vi "FGV Aufheizphase.vi"(0 "Status":T1, 7 "Error":bool, 9 "Aktiv/Inaktiv":u16, 11 "error in (no error)":errorcluster caption="Fehler (Eingang, kein Fehler)", 13 "Aktion":T2=enum."lesen") -> (4 "Aufheizphase":bool, 8 "Status":T1, 15 "error out":errorcluster caption="Fehler (Ausgang)")   [LabVIEW 2020, in "allgemeine Sub-VIs.lvlib"]
uses:
  allgemeine Sub-VIs.lvlib
  Aktion FGV Aufheizphase.ctl
  AufheizphaseCluster.ctl
  Funktionstasten/Funktionstasten-Aktion.ctl
  Funktionstasten/Zustaende.ctl
  Funktionstasten/Funktionstasten.lvlib
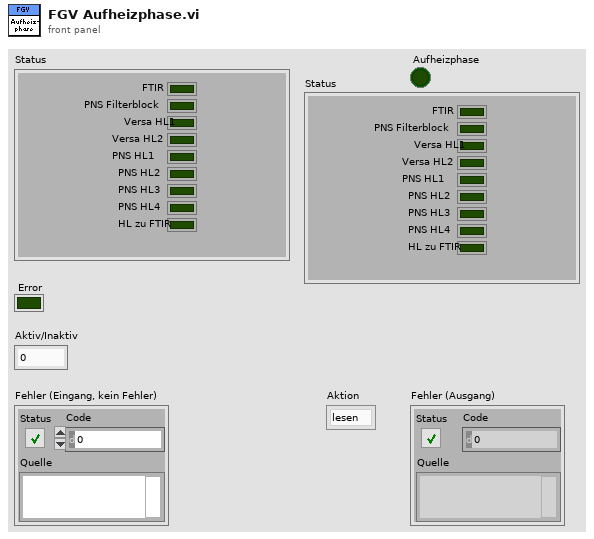
[diagram p1: front panel]
types:
  T1 = typedef "allgemeine Sub-VIs.lvlib/AufheizphaseCluster.ctl" = cluster{"FTIR":bool, "PNS Filterblock":bool, "Versa HL1":bool, "Versa HL2":bool, "PNS HL1":bool, "PNS HL2":bool, "PNS HL3":bool, "PNS HL4":bool, "HL zu FTIR":bool}
  T2 = typedef "allgemeine Sub-VIs.lvlib/Aktion FGV Aufheizphase.ctl" = enum16{"init", "lesen", "PNS Filterblock", "PNS HL1", "PNS HL2", "PNS HL3", "PNS HL4", "FTIR Messzelle", "HL 1", "HL 2", "HL zu FTIR", "auswerten"}
  T3 = typedef "Funktionstasten.lvlib/Zustaende.ctl" = enum16{"Standby", "Pause", "Eco", "Messen", "Kalibrieren", "Spülen Filter", "Spülen Leitung", "Umgebungsluft", "0-Gas", "Cal-Gas", "CG zu PNS", "-------------", "Init 1", "Init 2", "Init 3", "Init 4", "Messen vorbereiten", "Messen durchführen", "Exit"}
  T4 = typedef "Funktionstasten.lvlib/Funktionstasten-Aktion.ctl" = enum16{"Initialisieren", "Zustand setzen", "Taste gedrückt", "Fehler speichern", "Lesen", "Manuell", "Remote", "Bitparallel", "Samplepoint", "Zeit Prüfen", "reset Umschalten"}
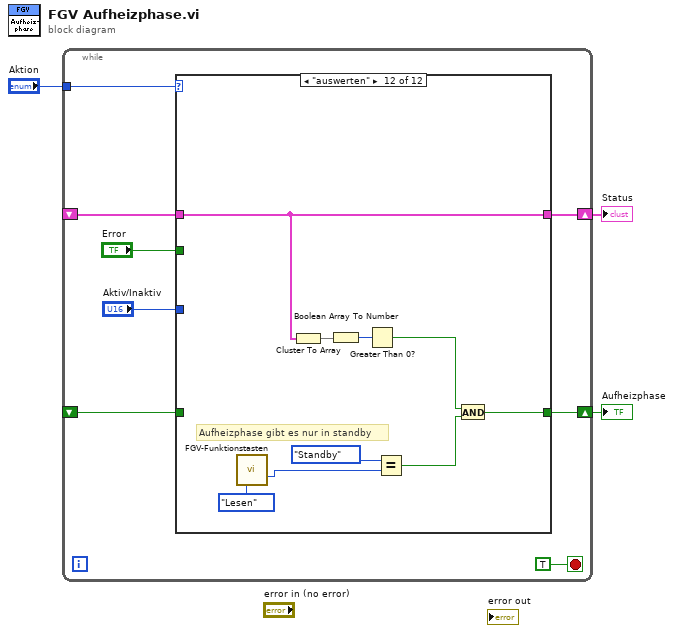
[diagram p0: block diagram]
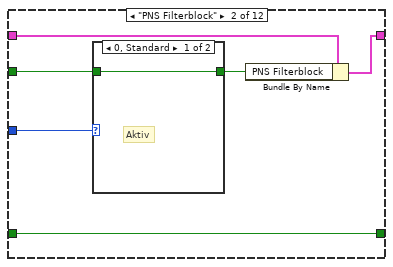
[diagram p3: hidden frame]
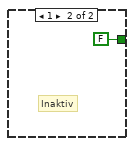
[diagram p4: hidden frame]
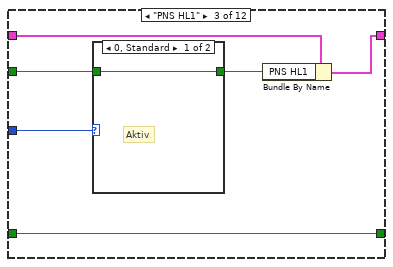
[diagram p5: hidden frame]
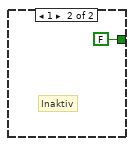
[diagram p6: hidden frame]
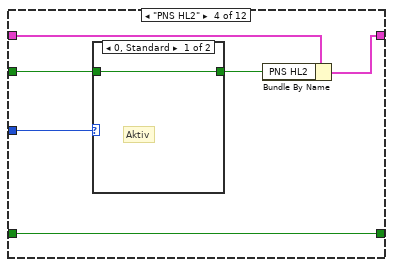
[diagram p7: hidden frame]
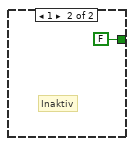
[diagram p8: hidden frame]
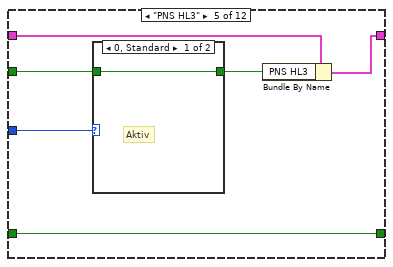
[diagram p9: hidden frame]
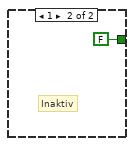
[diagram p10: hidden frame]
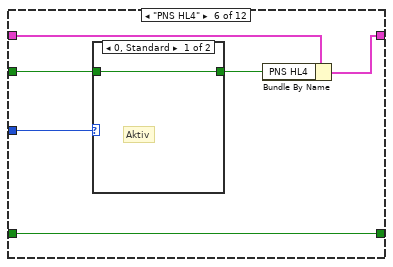
[diagram p11: hidden frame]
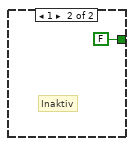
[diagram p12: hidden frame]
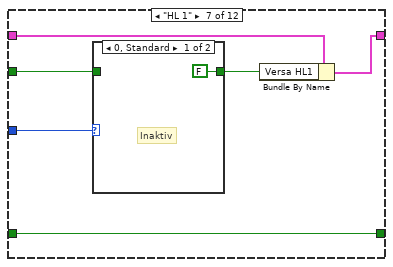
[diagram p13: hidden frame]
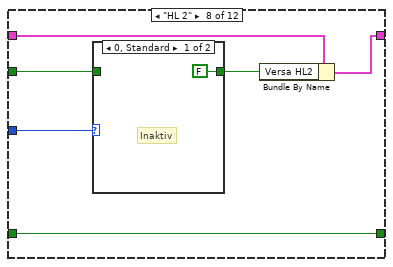
[diagram p15: hidden frame]
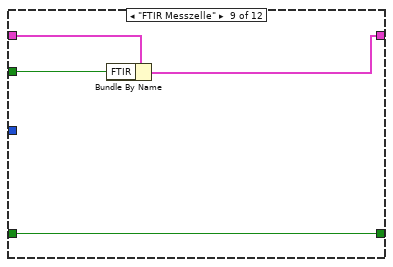
[diagram p17: hidden frame]
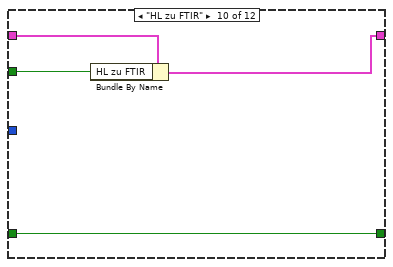
[diagram p18: hidden frame]
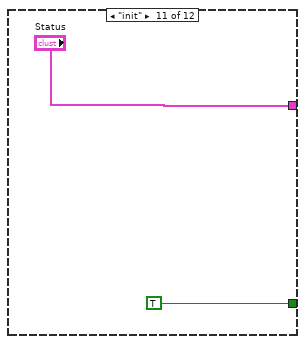
[diagram p19: hidden frame]
diagram:
  n1 = while {
    tunnel: "Aktion" -> [w10]
    shift-right: [w9] -> w1
    shift-left: _ -> [w8]
    shift-right: [w5] -> w2
    shift-left: _ -> [w4]
    stop <- TRUE stop-if-true
    n2 = case shown="\"auswerten\"" w10 {
      tunnel: [w13 w18 w26 w34 w42 w50 w58 w66 w72 w76 "Status" w88] -> w9
      tunnel: w8 -> [w13 w19 w27 w35 w43 w51 w59 w67 w73 w77 _ w88]
      tunnel: "Error" -> [_ w16 w24 w32 w40 w48 w56 w64 w71 w75 _ _]
      tunnel: "Aktiv/Inaktiv" -> [_ w17 w25 w33 w41 w49 w57 w65 _ _ _ _]
      tunnel: [w12 w14 w22 w30 w38 w46 w54 w62 w70 w74 TRUE w81] -> w5
      tunnel: w4 -> [w12 w14 w22 w30 w38 w46 w54 w62 w70 w74 _ _]
      frame "lesen", Default {
      }
      frame "PNS Filterblock" {
        n3 = case shown="0, Standard" w17 {
          tunnel: w16 -> [w20 _]
          tunnel: [w20 FALSE ("Error")] -> w15
          frame 0, Default {
            # "Aktiv"
          }
          frame 1 {
            # "Inaktiv"
          }
        }
        n4 = Bundle By Name(cluster=w19, "PNS Filterblock"=w15) -> (w18:T1)
      }
      frame "PNS HL1" {
        n5 = case shown="0, Standard" w25 {
          tunnel: w24 -> [w28 _]
          tunnel: [w28 FALSE ("Error")] -> w23
          frame 0, Default {
            # "Aktiv"
          }
          frame 1 {
            # "Inaktiv"
          }
        }
        n6 = Bundle By Name(cluster=w27, "PNS HL1"=w23) -> (w26:T1)
      }
      frame "PNS HL2" {
        n7 = case shown="0, Standard" w33 {
          tunnel: w32 -> [w36 _]
          tunnel: [w36 FALSE ("Error")] -> w31
          frame 0, Default {
            # "Aktiv"
          }
          frame 1 {
            # "Inaktiv"
          }
        }
        n8 = Bundle By Name(cluster=w35, "PNS HL2"=w31) -> (w34:T1)
      }
      frame "PNS HL3" {
        n9 = case shown="0, Standard" w41 {
          tunnel: w40 -> [w44 _]
          tunnel: [w44 FALSE ("Error")] -> w39
          frame 0, Default {
            # "Aktiv"
          }
          frame 1 {
            # "Inaktiv"
          }
        }
        n10 = Bundle By Name(cluster=w43, "PNS HL3"=w39) -> (w42:T1)
      }
      frame "PNS HL4" {
        n11 = case shown="0, Standard" w49 {
          tunnel: w48 -> [w52 _]
          tunnel: [w52 FALSE ("Error")] -> w47
          frame 0, Default {
            # "Aktiv"
          }
          frame 1 {
            # "Inaktiv"
          }
        }
        n12 = Bundle By Name(cluster=w51, "PNS HL4"=w47) -> (w50:T1)
      }
      frame "HL 1" {
        n13 = case shown="0, Standard" w57 {
          tunnel: w56 -> [_ w61]
          tunnel: [FALSE ("Error") w61] -> w55
          frame 0, Default {
            # "Inaktiv"
          }
          frame 1 {
            # "Aktiv"
          }
        }
        n14 = Bundle By Name(cluster=w59, "Versa HL1"=w55) -> (w58:T1)
      }
      frame "HL 2" {
        n15 = case shown="0, Standard" w65 {
          tunnel: w64 -> [_ w69]
          tunnel: [FALSE ("Error") w69] -> w63
          frame 0, Default {
            # "Inaktiv"
          }
          frame 1 {
            # "Aktiv"
          }
        }
        n16 = Bundle By Name(cluster=w67, "Versa HL2"=w63) -> (w66:T1)
      }
      frame "FTIR Messzelle" {
        n17 = Bundle By Name(cluster=w73, "FTIR"=w71) -> (w72:T1)
      }
      frame "HL zu FTIR" {
        n18 = Bundle By Name(cluster=w77, "HL zu FTIR"=w75) -> (w76:T1)
      }
      frame "init" {
      }
      frame "auswerten" {
        # "Aufheizphase gibt es nur in standby"
        n19 = call "FGV-Funktionstasten.vi"("Aktion"=Funktionstasten-Aktion."Lesen") -> ("ausgewählte Funktion"=w83:T3)  [unwired: 7 in, 7 out]
        n20 = Cluster To Array(cluster=w88) -> (array=w87:bool[])
        n21 = Boolean Array To Number(Boolean array=w87) -> (number=w86:u32)
        n22 = Greater Than 0?(x=w86) -> (x > 0?=w85:bool)
        n23 = Equal?(x=Zustaende."Standby", y=w83) -> (x = y?=w80:bool)
        n24 = And(x=w85, y=w80) -> (x .and. y?=w81:bool)
      }
    }
  }
  "Aufheizphase" <- w2
  "Status" <- w1
